vi "Function.vi"(8 "error in (no error)":errorcluster, 9 "Bool B":T1, 10 "Bool A":T1, 11 "AND in":refnum<class "NAND_U64.lvclass">) -> (0 "error out":errorcluster, 2 "Result":T1, 3 "AND out":refnum<class "NAND_U64.lvclass">)   [LabVIEW 2021, in "NAND_U64.lvclass"]
uses:
  NAND_U64.lvclass
  Type.ctl
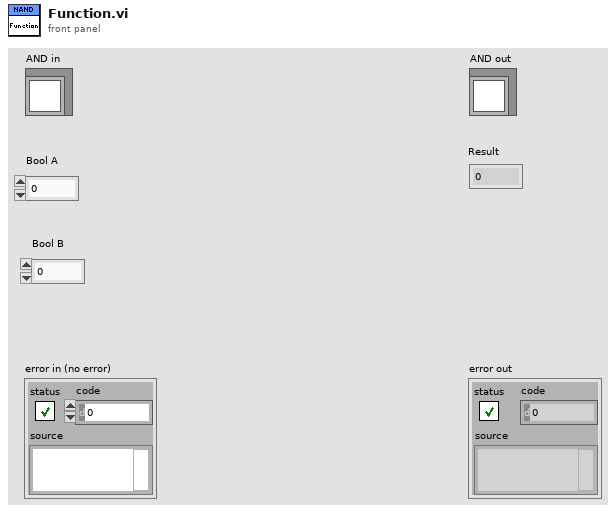
[diagram p1: front panel]
types:
  T1 = typedef "NAND_U64.lvclass/Type.ctl" = u64
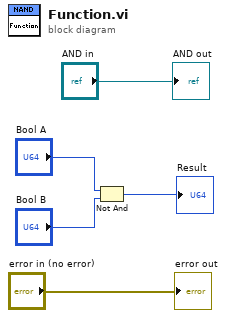
[diagram p0: block diagram]
diagram:
  n1 = Not And(1:"Bool B", 2:"Bool A") -> (0:→"Result":T1)
  "error out" <- "error in (no error)"
  "AND out" <- "AND in"
